vi "Edit Line.vi"(8 "error in":errorcluster, 10 "Line Name":string, 11 "References":T1) -> (0 "error out":errorcluster, 2 "change?":bool)   [LabVIEW 2015, in "SystemLink File editor node.lvclass"]
doc: "This VI edits the properties of a line. It will unlink channels and tags and create new links to channels and tags."
uses:
  SystemLink File editor node.lvclass
  <vilib>/NI/DCAF/Tag Editor Core/Configuration Editor/Classes/Engine Parent/Engine Parent Editor Node.lvclass
  module/configuration/SystemLink File configuration.lvclass
  <vilib>/NI/Configuration Framework/serializable configuration/NISE_CEF_serializable configuration.lvclass
  <vilib>/NI/DCAF/Tag Editor Core/Configuration Editor/Classes/Module editor node/module editor node.lvclass
  <vilib>/NI/DCAF/Tag Editor Core/Table API/Table Manager/object ref.ctl
  <vilib>/NI/DCAF/Tag Editor Core/Table API/Table Manager/Table Manager.lvclass
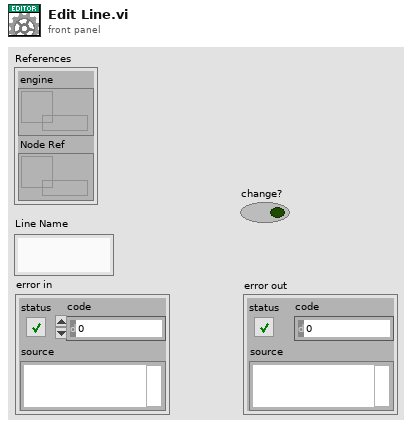
[diagram p1: front panel]
types:
  T1 = typedef "Table Manager.lvlib/Table Manager.lvclass/object ref.ctl" = cluster{"engine":refnum<data-value>, "Node Ref":refnum<data-value>}
  T2 = typedef "SystemLink File configuration.lvclass/Line.ctl" = cluster{"channel":refnum<class "TBM channel.lvclass">, "Data Tag Type":T3}
  T3 = typedef "SystemLink File configuration.lvclass/Data Tag Type.ctl" = enum16{"Double", "Single", "I32", "I16", "I8", "U64", "U32", "U16", "U8", "Boolean", "String", "Timestamp"}
  T4 = typedef "SystemLink File editor node.lvclass/Mappings.ctl" = cluster{"Line":T2, "Maps":T5[]}
  T5 = typedef "SystemLink File editor node.lvclass/Map.ctl" = cluster{"channel":refnum<class "TBM channel.lvclass">, "tag name":string}
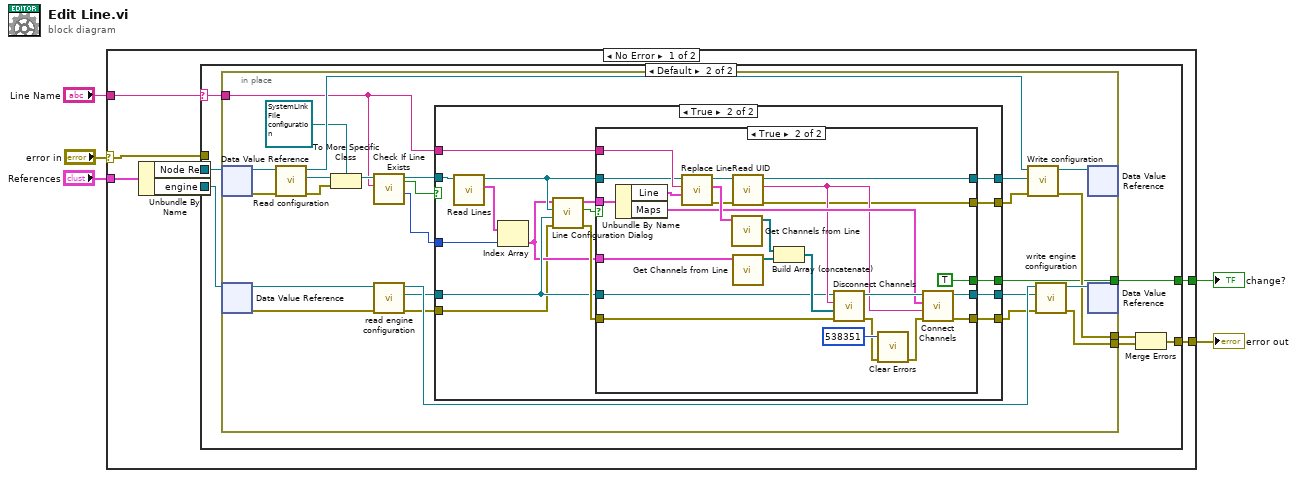
[diagram p0: block diagram]
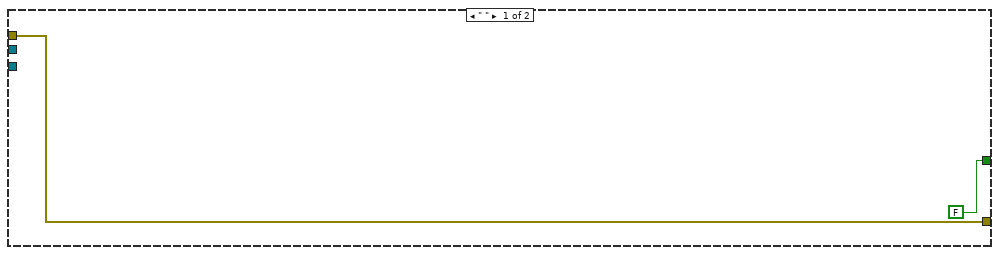
[diagram p2: hidden frame]
diagram:
  n1 = case shown="No Error" "error in" {
    selector: "error in" -> [w6 w93]
    tunnel: "References" -> [w10 _]
    tunnel: "Line Name" -> [w7 _]
    tunnel: [w9 w93] -> w2
    tunnel: [w8 _] -> w1
    frame No Error {
      n2 = Unbundle By Name(w10) -> ("Node Ref"=w12:refnum<data-value>, "engine"=w11:refnum<data-value>)
      n3 = case shown="Default" w7 {
        selector: w7 -> [_ w15]
        tunnel: w12 -> [_ w21]
        tunnel: w11 -> [_ w20]
        tunnel: [w13 w17] -> w9
        tunnel: [FALSE ("change?") w16] -> w8
        tunnel: w6 -> [w13 _]
        frame " " {
        }
        frame Default {
          n4 = in-place {
            in-place-border: [w28] -> w19
            in-place-border: [w43] -> w18
            in-place-border: [w27] -> w16
            in-place-border: w15 -> [w33]
            n5 = in-place-dvr #1(w21) -> (w40:refnum<class "module editor node.lvclass">, w34:errorcluster)
            n6 = in-place-dvr #2(w20) -> (w46:refnum<class "Engine Parent Editor Node.lvclass">, w45:errorcluster)
            n7 = call-dynamic "Read configuration.vi"("error in"=w34, "NISE_CEF_serializable node in"=w40) -> ("error out"=w37:errorcluster, "configuration"=w38:refnum<class "NISE_CEF_serializable configuration.lvclass">, "NISE_CEF_serializable node out"=w39:refnum<class "module editor node.lvclass">)  [unwired: 7 in]
            n8 = To More Specific Class(target class=refnum<class "SystemLink File configuration.lvclass"> refnum ("tag bus configurable plugin module configuration"), reference=w38, error in=w37) -> (specific class reference=w35:refnum<class "SystemLink File configuration.lvclass">)  [unwired: 1 out]
            n9 = call-dynamic "Check If Line Exists.vi"("Name to Locate"=w33, "SystemLin Tag Module configuration in"=w35) -> ("Index"=w30:i32, "SystemLin Tag Module configuration out"=w31:refnum<class "SystemLink File configuration.lvclass">, "Found?"=w25:bool)  [unwired: 5 in, 2 out]
            n10 = call <vilib>:"read engine configuration.vi"("error in"=w45, "Engine Parent Editor Node in"=w46) -> ("error out"=w22:errorcluster, "engine configuration"=w29:refnum<class "engine configuration.lvclass">, "Engine Parent Editor Node out"=w42:refnum<class "Engine Parent Editor Node.lvclass">)  [unwired: 7 in]
            n11 = case shown="True" w25 {
              tunnel: w31 -> [w49 w63]
              tunnel: w29 -> [w48 w54]
              tunnel: w33 -> [_ w65]
              tunnel: [w49 w58] -> w32
              tunnel: w30 -> [_ w60]
              tunnel: [_ w56] -> w27
              tunnel: [w48 w55] -> w26
              tunnel: [_ w53] -> w24
              tunnel: [w47 w51] -> w23
              tunnel: w22 -> [w47 w50]
              frame False {
              }
              frame True {
                n12 = call "Read Lines.vi"("SystemLin Tag Module configuration in"=w63) -> ("Lines"=w61:T2[], "SystemLin Tag Module configuration out"=w62:refnum<class "SystemLink File configuration.lvclass">)  [unwired: 8 in, 1 out]
                n13 = Index Array(array=w61, index=w60) -> (element=w52:T2)
                n14 = call "Line Configuration Dialog.vi"("error in"=w50, "engine configuration in"=w54, "tag bus configurable plugin module configuration"=w62, "Line"=w52) -> ("error out"=w64:errorcluster, "changed"=w57:bool, "Mappings out"=w59:T4)  [unwired: 4 in, 1 out]
                n15 = case shown="True" w57 {
                  tunnel: w65 -> [_ w92]
                  tunnel: w54 -> [w67 w76]
                  tunnel: w64 -> [w66 w91]
                  tunnel: w62 -> [w68 w88]
                  tunnel: w59 -> [_ w87]
                  tunnel: [w68 w85] -> w58
                  tunnel: [_ TRUE ("change?")] -> w56
                  tunnel: [w67 w80] -> w55
                  tunnel: [_ w71] -> w53
                  tunnel: w52 -> [_ w70]
                  tunnel: [w66 w69] -> w51
                  frame False {
                  }
                  frame True {
                    n16 = Unbundle By Name(w87) -> ("Line"=w86:T2, "Maps"=w83:T5[])
                    n17 = call "Replace Line.vi"("New Line"=w86, "Line Name"=w92, "SystemLin Tag Module configuration in"=w88) -> ("error out"=w72:errorcluster, "Old Line"=w89:T2, "SystemLin Tag Module configuration out"=w90:refnum<class "SystemLink File configuration.lvclass">)  [unwired: 6 in]
                    n18 = call "Get Channels from Line.vi"("Line"=w89) -> ("Channels"=w79:refnum<class "TBM channel.lvclass">[])  [unwired: 10 in]
                    n19 = call <vilib>:"Read UID.vi"("error in"=w72, "configuration in"=w90) -> ("error out"=w71:errorcluster, "instance id"=w82:string, "configuration out"=w85:refnum<class "SystemLink File configuration.lvclass">)  [unwired: 7 in]
                    n20 = call "Get Channels from Line.vi"("Line"=w70) -> ("Channels"=w78:refnum<class "TBM channel.lvclass">[])  [unwired: 10 in]
                    n21 = Build Array (concatenate)(w79, w78) -> (w77:refnum<class "TBM channel.lvclass">[])
                    n22 = call "Disconnect Channels.vi"("error in (no error)"=w91, "Deleted Channels"=w77, "instance id"=w82, "Engine Configuration in"=w76) -> ("error out"=w74:errorcluster, "Engine Configuration out"=w84:refnum<class "engine configuration.lvclass">)  [unwired: 6 in]
                    n23 = call <vilib>:"Clear Errors.vi"("error in (no error)"=w74, "specific error code to clear (0: all)"=538351) -> ("error out"=w73:errorcluster)  [unwired: 4 in, 1 out]
                    n24 = call "Connect Channels.vi"("error in (no error)"=w73, "instance id"=w82, "Maps"=w83, "Engine Configuration in"=w84) -> ("error out"=w69:errorcluster, "Engine Configuration out"=w80:refnum<class "engine configuration.lvclass">)  [unwired: 6 in]
                  }
                }
              }
            }
            n25 = call-dynamic "Write configuration.vi"("error in"=w24, "configuration"=w32, "NISE_CEF_serializable node in"=w39) -> ("error out"=w28:errorcluster, "NISE_CEF_serializable node out"=w41:refnum<class "module editor node.lvclass">)  [unwired: 7 in]
            n26 = call <vilib>:"write engine configuration.vi"("error in"=w23, "engine configuration"=w26, "Engine Parent Editor Node in"=w42) -> ("error out"=w43:errorcluster, "Engine Parent Editor Node out"=w44:refnum<class "Engine Parent Editor Node.lvclass">)  [unwired: 7 in]
            n27 = in-place-dvr #1(w41) -> ()  [unwired: 2 out]
            n28 = in-place-dvr #2(w44) -> ()  [unwired: 2 out]
          }
          n29 = Merge Errors(w19, w18) -> (w17:errorcluster)
        }
      }
    }
    frame Error {
    }
  }
  "change?" <- w1
  "error out" <- w2
